vi "Kill Process.vi"(8 "Error In":errorcluster, 11 "Process Name":string) -> (0 "Error Out":errorcluster)   [LabVIEW 2020, in "LMH-Toolbox.lvlib"]
doc: "Kill a process by name."
uses:
  LMH-Toolbox.lvlib
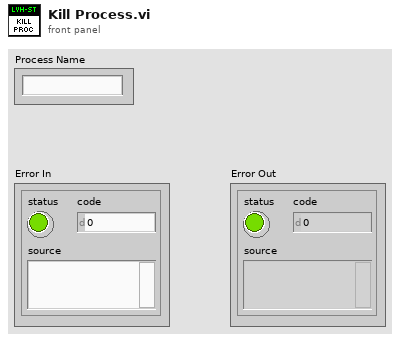
[diagram p1: front panel]
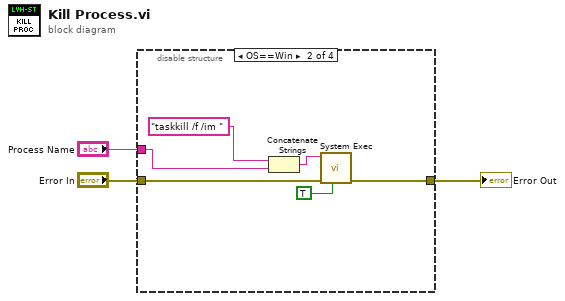
[diagram p0: block diagram]
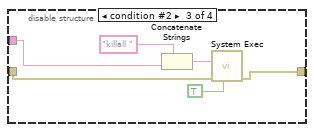
[diagram p3: hidden frame]
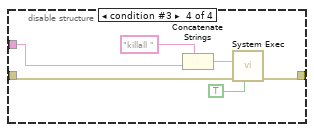
[diagram p4: hidden frame]
diagram:
  n1 = disable-structure shown="OS==Win" {
    disable-tunnel: [w4 w7 w14 w19] -> w3
    disable-tunnel: "Error In" -> [w4 w8 w15 w18]
    disable-tunnel: "Process Name" -> [_ w10 w12 w17]
    frame condition #0 {
    }
    frame condition #1 (active) {
      n2 = Concatenate Strings("taskkill /f /im ", w10) -> (w5:string)
      n3 = call <vilib>:"System Exec.vi"("run minimized? (F)"=TRUE, "error in (no error)"=w8, "command line"=w5) -> ("error out"=w7:errorcluster)  [unwired: 5 in, 3 out]
    }
    frame condition #2 {
      n4 = Concatenate Strings("killall ", w12) -> (w13:string)
      n5 = call <vilib>:"System Exec.vi"("run minimized? (F)"=TRUE, "error in (no error)"=w15, "standard input"=w13) -> ("error out"=w14:errorcluster)  [unwired: 5 in, 3 out]
    }
    frame condition #3 {
      n6 = Concatenate Strings("killall ", w17) -> (w21:string)
      n7 = call <vilib>:"System Exec.vi"("run minimized? (F)"=TRUE, "error in (no error)"=w18, "standard input"=w21) -> ("error out"=w19:errorcluster)  [unwired: 5 in, 3 out]
    }
  }
  "Error Out" <- w3
